vi "FileLoaderAuto.vi"(9 "index":i32) -> (1 "coerced index":i32, 3 "Auto Array":dbl[][](array[numeric]) format="%0.3f")   [LabVIEW 2013]
uses:
  Robot Global Data.vi
  <vilib>/Utility/file.llb/Read From Spreadsheet File (DBL).vi
panel:
  out "String":string
  out "Files":string
  out "Auto Array":dbl[][](array[numeric]) format="%0.3f"
  in  "File Name":string
  # "The Working One"
  # "Currently Disabled because it is old code"
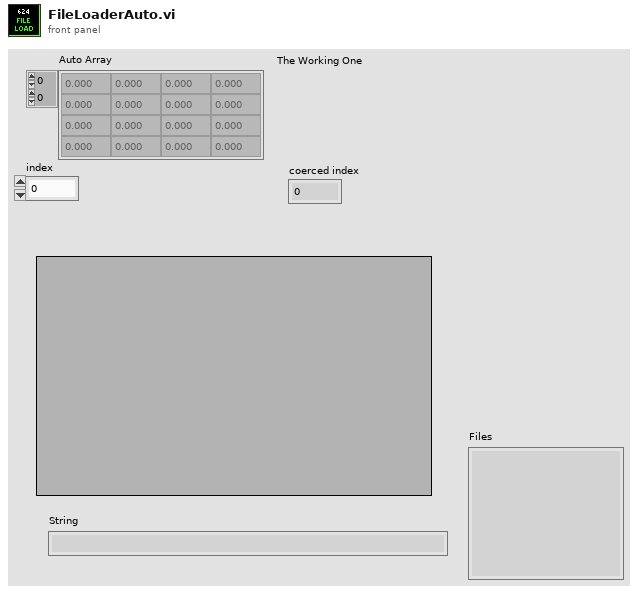
[diagram p1: front panel]
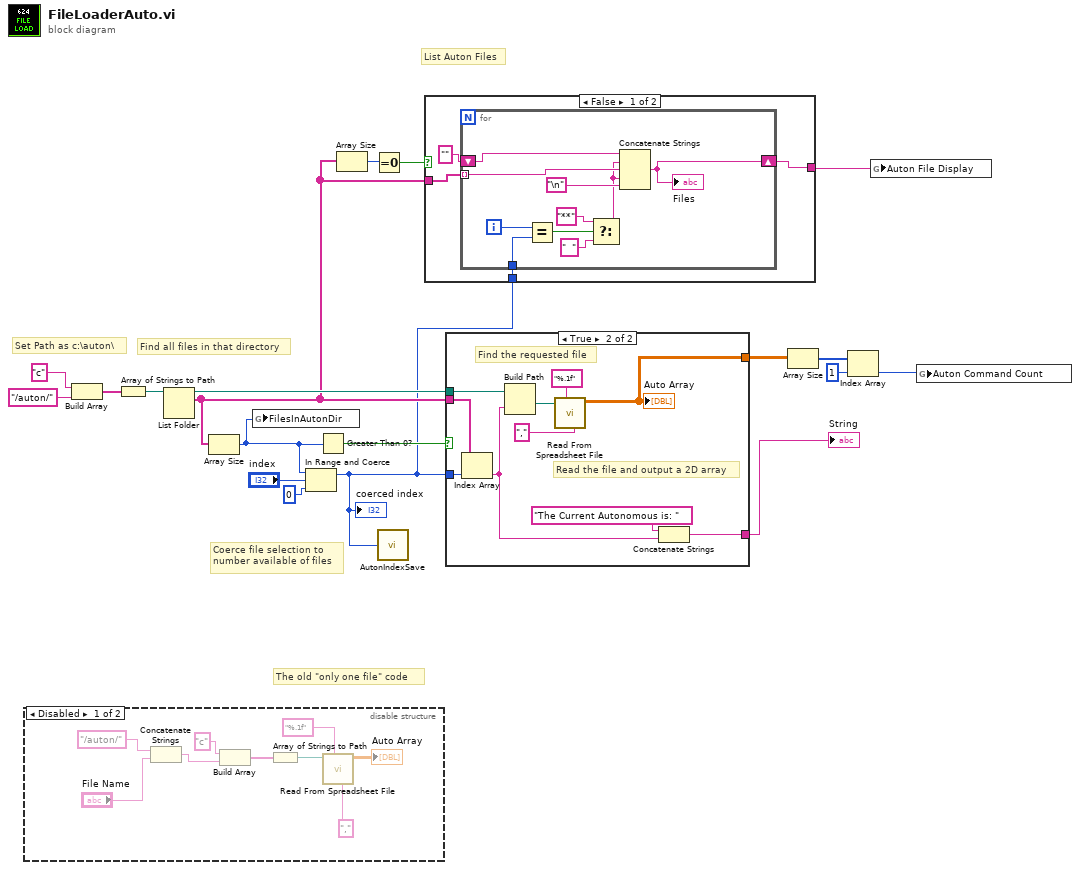
[diagram p0: block diagram]
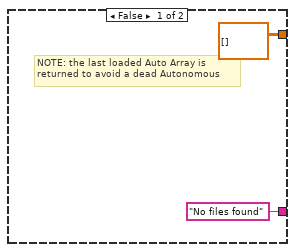
[diagram p2: hidden frame]
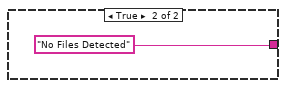
[diagram p3: hidden frame]
diagram:
  # "List Auton Files"
  # "Coerce file selection to\nnumber available of files"
  # "Find all files in that directory"
  # "Set Path as c:\\auton\\"
  # "The old \"only one file\" code"
  n1 = disable-structure shown="Disabled" {
    frame Disabled {
      n2 = Concatenate Strings("/auton/" ("string"), "File Name") -> (w26:string)
      n3 = Build Array("c" ("element"), w26) -> (w24:string[])
      n4 = Array of Strings to Path(0:w24) -> (2:w23:path)  [unwired: 1 in]
      n5 = call-poly <vilib>:"Read From Spreadsheet File.vi"("delimiter (\\t)"="," ("delimiter (\\t)"), "format (%.3f)"="%.1f", "file path (dialog if empty)"=w23) -> ("all rows"=→"Auto Array":dbl[][])  [unwired: 4 in, 4 out]
    }
    frame Enabled {
    }
  }
  n6 = Build Array("c" ("element"), "/auton/" ("string")) -> (w16:string[])
  n7 = Array of Strings to Path(0:w16) -> (2:w19:path)  [unwired: 1 in]
  n8 = List Folder(path=w19) -> (path out=w15:path, filenames=w8:string[])  [unwired: 3 in, 2 out]
  n9 = Array Size(array=w8) -> (size(s)=w12:i32)
  n10 = global write "Robot Global Data.vi" "FilesInAutonDir"(w12) -> ()
  n11 = In Range and Coerce(upper limit=w12, x="index", lower limit=0) -> (coerced(x)=w1:i32)  [unwired: 1 out]
  "coerced index" <- w1
  n12 = Greater Than 0?(x=w12) -> (x > 0?=w11:bool)
  n13 = Array Size(array=w8) -> (size(s)=w9:i32)
  n14 = Equal To 0?(x=w9) -> (x = 0?=w7:bool)
  n15 = call "AutonIndexSave.vi"("index"=w1) -> ()  [unwired: 1 in]
  n16 = case shown="False" w7 {
    tunnel: w1 -> [w31 _]
    tunnel: [w30 "No Files Detected"] -> w2
    tunnel: w8 -> [w29 _]
    frame False {
      n17 = for {
        shift-right: [w42] -> w30
        shift-left: "" -> [w34]
        tunnel: w29 -> [w41] mode=indexing
        tunnel: w31 -> [w39]
        i -> [w40]
        n18 = Equal?(x=w40, y=w39) -> (x = y?=w38:bool)
        n19 = Select(t="**", s=w38, f="  ") -> (s? t:f=w33:string)
        n20 = Concatenate Strings(w34, w33, w41, w33, "\n") -> (w42:string)
        "Files" <- w42
      }
    }
    frame True {
    }
  }
  n21 = case shown="True" w11 {
    tunnel: w15 -> [_ w51]
    tunnel: w8 -> [_ w48]
    tunnel: w1 -> [_ w47]
    tunnel: ["No files found" w46] -> w10
    tunnel: [dbl[][] [] ("all rows") w53] -> w6
    frame False {
      # "NOTE: the last loaded Auto Array is\nreturned to avoid a dead Autonomous"
    }
    frame True {
      # "Read the file and output a 2D array"
      # "Find the requested file"
      n22 = Index Array(array=w48, index=w47) -> (element=w49:string)
      n23 = Build Path(base path=w51, name or relative path=w49) -> (appended path=w52:path)
      n24 = call-poly <vilib>:"Read From Spreadsheet File.vi"("delimiter (\\t)"="," ("delimiter (\\t)"), "format (%.3f)"="%.1f", "file path (dialog if empty)"=w52) -> ("all rows"=w53:dbl[][])  [unwired: 4 in, 4 out]
      "Auto Array" <- w53
      n25 = Concatenate Strings("The Current Autonomous is: ", w49) -> (w46:string)
    }
  }
  "String" <- w10
  n26 = Array Size(array=w6) -> (size(s)=w5:i32[])
  n27 = Index Array(array=w5, index=1) -> (element=w3:i32)
  n28 = global write "Robot Global Data.vi" "Auton File Display"(w2) -> ()
  n29 = global write "Robot Global Data.vi" "Auton Command Count"(w3) -> ()
